vi "ReadWrite.Data.vi"(8 "error in (no error)":errorcluster, 10 "timeout ms":i32=100, 11 "Ref":refnum<data-value>) -> (0 "error out":errorcluster, 1 "Timeout?":bool, 2 "Data":dbl[](array[numeric]))   [LabVIEW 2015, in "Data Access API.lvlib" / "Data Access API.lvclass"]
uses:
  Data Access API.lvclass
  Data/ReadWrite/ReadWrite.lvclass
  Data/ReadWrite/ReadWrite.lvclass/ReadWrite.ctl
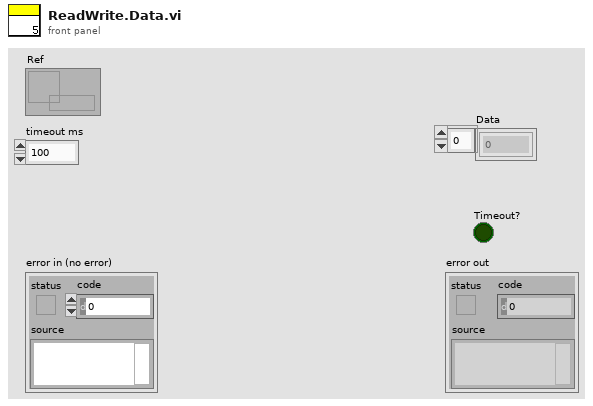
[diagram p1: front panel]
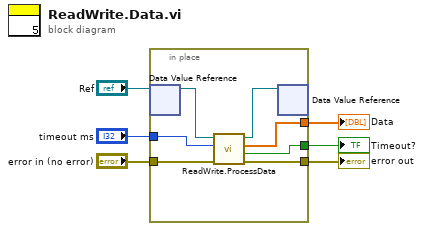
[diagram p0: block diagram]
diagram:
  n1 = in-place {
    in-place-border: "error in (no error)" -> [w11]
    in-place-border: [w10] -> w5
    in-place-border: "timeout ms" -> [w9]
    in-place-border: [w8] -> w2
    in-place-border: [w7] -> w1
    n2 = in-place-dvr #1("Ref") -> (w13:refnum<class "ReadWrite.lvclass">)  [unwired: 1 out]
    n3 = call "ReadWrite.ProcessData.vi"("error in (no error)"=w11, "timeout ms"=w9, "ReadWrite in"=w13) -> ("error out"=w10:errorcluster, "Timeout?"=w7:bool, "Values"=w8:dbl[], "ReadWrite out"=w12:refnum<class "ReadWrite.lvclass">)  [unwired: 5 in]
    n4 = in-place-dvr #1(w12) -> ()  [unwired: 2 out]
  }
  "error out" <- w5
  "Data" <- w2
  "Timeout?" <- w1
